vi "str_minuslast.vi"(1 "N":i32=1, 2 "String In":string) -> (6 "String Out":string)   [LabVIEW 2018]
doc: "Removes the last N characters from a string."
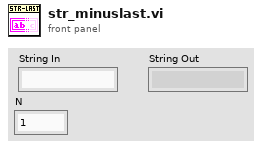
[diagram p1: front panel]
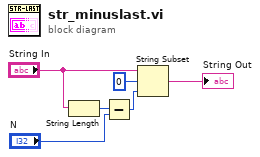
[diagram p0: block diagram]
diagram:
  n1 = String Length(string="String In") -> (length=w3:i32)
  n2 = Subtract(x=w3, y="N") -> (x-y=w2:i32)
  n3 = String Subset(string="String In", offset (0)=0, length (rest)=w2) -> (substring=→"String Out":string)
